vi "initiate.vi"(8 "error in (no error)":errorcluster, 11 "UI Port Address":u32=3005) -> (0 "error out":errorcluster, 3 "simple_html_chat_ui out":refnum<class "simple_html_chat_ui.lvclass">)   [LabVIEW 2020, in "simple_html_chat_ui.lvclass"]
uses:
  simple_html_chat_ui.lvclass
  simple_html_chat_ui.lvclass/simple_html_chat_ui.ctl
  ui/View.vi
  <vilib>/httpClient/LabVIEWHTTPClient.lvlib
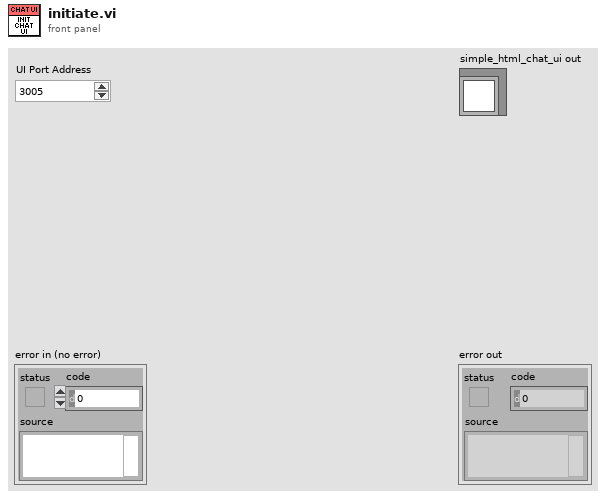
[diagram p1: front panel]
types:
  T1 = typedef "LabVIEWHTTPClient.lvlib/ClientHandle.ctl" = refnum<k1>
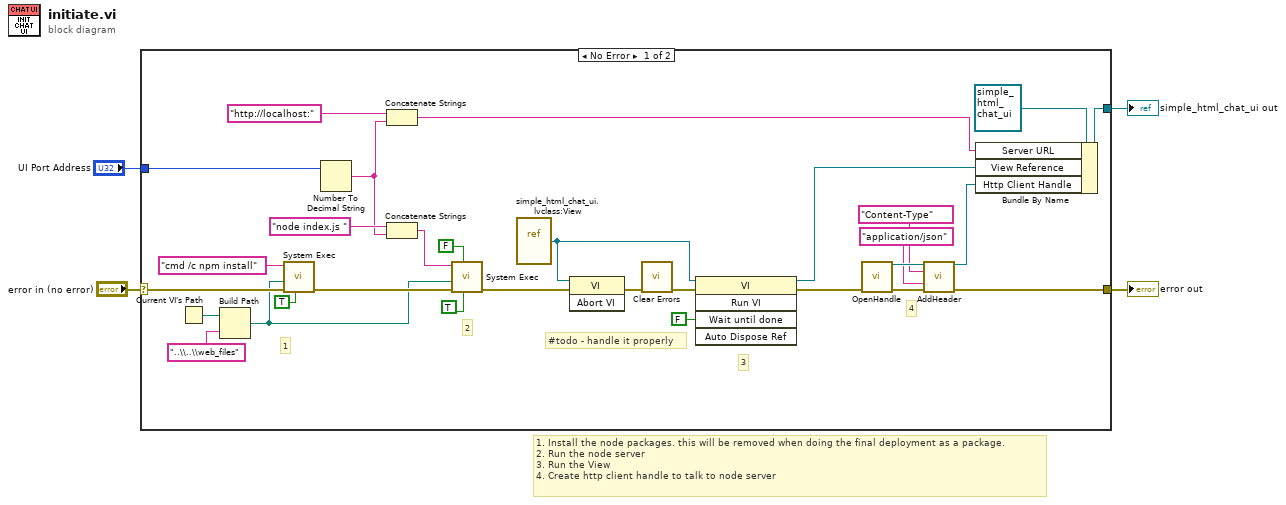
[diagram p0: block diagram]
diagram:
  # "1. Install the node packages. this will be removed when doing the final deployment as a package.\n2. Run the node server\n3. Run the View\n4. Create http client handle to talk to node server"
  n1 = case shown="No Error" "error in (no error)" {
    selector: "error in (no error)" -> [w33 w34]
    tunnel: [w17 w34] -> w3
    tunnel: [w27 _] -> w2
    tunnel: "UI Port Address" -> [w29 _]
    frame No Error {
      # "#todo - handle it properly"
      # "4"
      # "3"
      # "2"
      # "1"
      n2 = Current VI's Path() -> (path=w32:path)
      n3 = Build Path(base path=w32, name or relative path="..\\..\\web_files") -> (appended path=w15:path)
      n4 = call <vilib>:"System Exec.vi"("run minimized? (F)"=TRUE, "error in (no error)"=w33, "working directory"=w15, "command line"="cmd /c npm install") -> ("error out"=w30:errorcluster)  [unwired: 4 in, 3 out]
      n5 = Number To Decimal String(number=w29) -> (decimal integer string=w6:string)  [unwired: 1 in]
      n6 = Concatenate Strings("http://localhost:", w6) -> (w12:string)
      n7 = Concatenate Strings("node index.js " ("command line"), w6) -> (w5:string)
      n8 = call <vilib>:"System Exec.vi"("run minimized? (F)"=TRUE, "wait until completion? (T)"=FALSE, "error in (no error)"=w30, "working directory"=w15, "command line"=w5) -> ("error out"=w26:errorcluster)  [unwired: 3 in, 3 out]
      n9 = vi-ref "simple_html_chat_ui.lvclass:View.vi"() -> (w9:refnum<vi>)
      n10 = invoke class="VI" method="Abort VI"(reference=w9) -> ()  [unwired: 2 in, 3 out]
      n11 = call <vilib>:"Clear Errors.vi"("error in (no error)"=w26) -> ("error out"=w8:errorcluster)  [unwired: 5 in, 1 out]
      n12 = invoke class="VI" method="Run VI"(reference=w9, error in=w8, "Wait until done"=FALSE ("Wait Until Done")) -> (reference out=w24:refnum<vi>, error out=w23:errorcluster)  [unwired: 2 in, 3 out]
      n13 = call <vilib>:"OpenHandle.vi"("error in (no error)"=w23) -> ("client handle out"=w21:T1, "error out"=w20:errorcluster)  [unwired: 13 in]
      n14 = call <vilib>:"AddHeader.vi"("client handle"=w21, "header"="Content-Type", "value"="application/json", "error in (no error)"=w20) -> ("client handle out"=w16:T1, "error out"=w17:errorcluster)  [unwired: 10 in]
      n15 = Bundle By Name(cluster=refnum<class "simple_html_chat_ui.lvclass"> refnum ("simple_html_chat_ui in"), "Server URL"=w12, "View Reference"=w24, "Http Client Handle"=w16) -> (w27:refnum<class "simple_html_chat_ui.lvclass">)
    }
    frame Error {
    }
  }
  "error out" <- w3
  "simple_html_chat_ui out" <- w2
